vi "Com_SECS Equipment _Release.vi"(8 "error in":errorcluster, 11 "Buffer Data":T1) -> (0 "error out":errorcluster)   [LabVIEW 2016]
uses:
  Data Def/Com_SECS Equipment _Buffer Data.ctl
  Data Def/Com_SECS Equipment _Connection Setting.ctl
  Data Def/Com_SECS Equipment _Timeout Setting.ctl
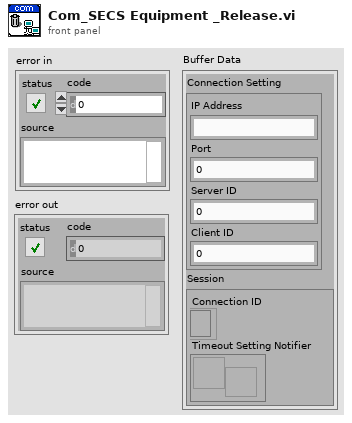
[diagram p1: front panel]
types:
  T1 = typedef "Com_SECS Equipment _Buffer Data.ctl" = cluster{"Connection Setting":T2, "Session":cluster{"Connection ID":refnum<k5>, "Timeout Setting Notifier":refnum<notifier>}}
  T2 = typedef "Com_SECS Equipment _Connection Setting.ctl" = cluster{"IP Address":string, "Port":u16, "Server ID":u16, "Client ID":u16}
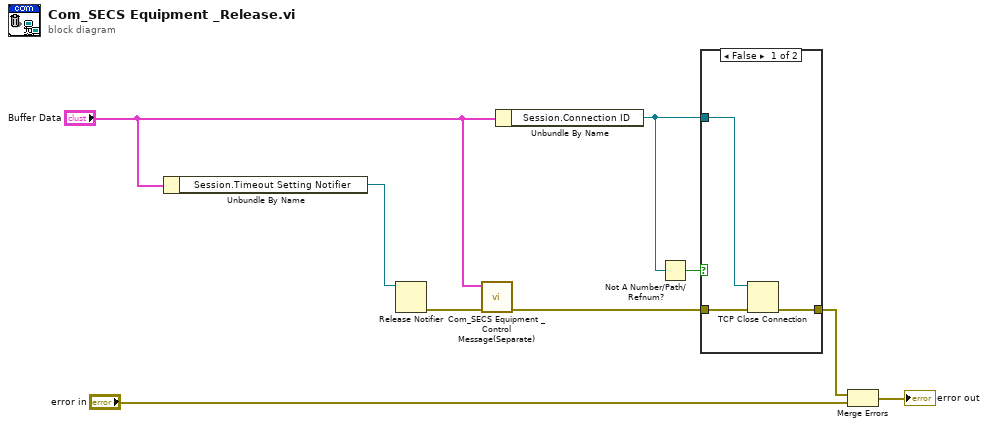
[diagram p0: block diagram]
diagram:
  n1 = Unbundle By Name("Buffer Data") -> ("Session.Timeout Setting Notifier"=w7:refnum<notifier>)
  n2 = Release Notifier(notifier=w7) -> (error out=w6:errorcluster)  [unwired: 2 in, 2 out]
  n3 = call "Com_SECS Equipment _Control Message(Separate).vi"("error in"=w6, "Buffer Data In"="Buffer Data") -> ("error out"=w1:errorcluster)  [unwired: 8 in, 1 out]
  n4 = Unbundle By Name("Buffer Data") -> ("Session.Connection ID"=w8:refnum<k5>)
  n5 = Not A Number/Path/Refnum?(number/path/refnum=w8) -> (NaN/Path/Refnum?=w9:bool)
  n6 = case shown="False" w9 {
    tunnel: w8 -> [w12 _]
    tunnel: w1 -> [w10 w13]
    tunnel: [w11 w13] -> w3
    frame False {
      n7 = TCP Close Connection(connection ID=w12, error in (no error)=w10) -> (error out=w11:errorcluster)  [unwired: 1 in, 1 out]
    }
    frame True {
    }
  }
  n8 = Merge Errors(w3, "error in") -> (→"error out":errorcluster)
